vi "Test 2 Map number Multiple inputs.vi"(8 "error in (no error)":errorcluster, 11 "Test Case In":refnum<class "Day 5 Test.lvclass">) -> (0 "error out":errorcluster, 3 "Test Case Out":refnum<class "Day 5 Test.lvclass">)   [LabVIEW 2020, in "Day 5 Test.lvclass"]
uses:
  Day 5 Test.lvclass
  C:/Program Files (x86)/National Instruments/LabVIEW 2020/vi.lib/Astemes/LUnit/Test Case.lvclass
  <vilib>/Astemes/LUnit/Test Case.lvclass/Test Case.ctl
  4993e8ee-a06a-463a-9684-69129f64d5ce.vi
  <vilib>/Astemes/LUnit/Append Pass Result.vi
  <vilib>/Astemes/LUnit/Append Fail Result.vi
  <vilib>/Astemes/LUnit/Describe Comparison.vi
  <vilib>/Astemes/LUnit/Compare Variants.vi
  <vilib>/Astemes/LUnit/Variant to string.vi
  <vilib>/Utility/Data Type/Get Type Information.vi
  <vilib>/Utility/LVClass/Get LV Class Name.vi
  Day 5 Test.lvclass/Day 5 Test.ctl
  Map/Map.lvclass
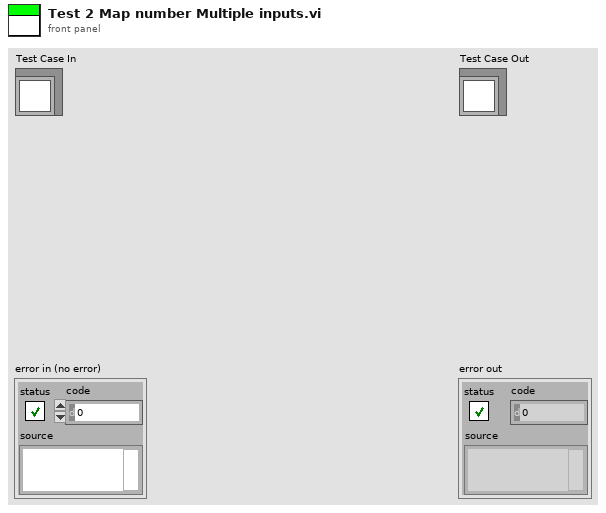
[diagram p1: front panel]
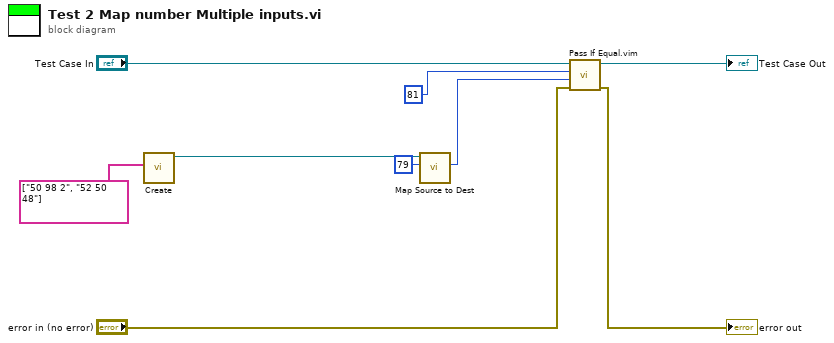
[diagram p0: block diagram]
diagram:
  n1 = call "Create.vi"("Input"=string[] ["50 98 2", "52 50 48"]) -> ("Map"=w5:refnum<class "Map.lvclass">)  [unwired: 9 in, 1 out]
  n2 = call "Map Source to Dest.vi"("Source"=u32 79, "Map in"=w5) -> ("Destination"=w3:u32)  [unwired: 7 in, 2 out]
  n3 = call "Pass If Equal.vim"("error in (no error)"="error in (no error)", "Actual"=w3, "Expected"=u32 81 ("Destination"), "LUnit Test Case In"="Test Case In") -> ("error out"=→"error out":errorcluster, "LUnit Test Case Out"=→"Test Case Out":refnum<class "Day 5 Test.lvclass">)  [unwired: 6 in]
